vi "Send Basic Command Packet.vi"(9 "Solenoid States":bool[](array[boolean]), 11 "Output Enable":bool) -> ()   [LabVIEW 2015]
uses:
  Control Packet - Basic.ctl
  Control Packet Type.ctl
  Packet Transmitter Action.ctl
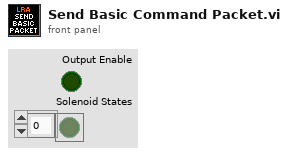
[diagram p1: front panel]
types:
  T1 = typedef "Packet Transmitter Action.ctl" = enum16{"Initialize", "Enqueue for Send", "Retrieve for Send"}
  T2 = typedef "Control Packet Type.ctl" = enum8{"Basic"}
  T3 = typedef "Control Packet - Basic.ctl" = cluster{"Solenoid Commands":bool[], "Output Enable":bool, "Timestamp":u32}
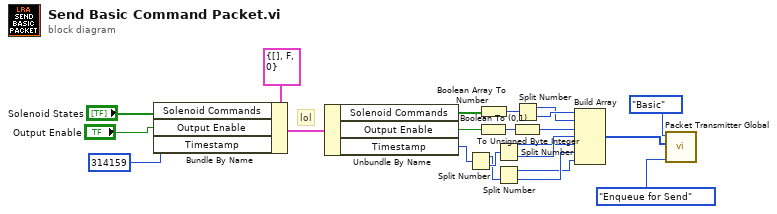
[diagram p0: block diagram]
diagram:
  # "lol"
  n1 = Bundle By Name(cluster=T3 {"Solenoid Commands"=[], "Output Enable"=FALSE, "Timestamp"=0} ("Cluster"), "Solenoid Commands"="Solenoid States", "Output Enable"="Output Enable", "Timestamp"=u32 314159) -> (w19:T3)
  n2 = Unbundle By Name(w19) -> ("Solenoid Commands"=w18:bool[], "Output Enable"=w17:bool, "Timestamp"=w11:u32)
  n3 = Split Number(x=w11) -> (hi(x)=w9:u16, lo(x)=w10:u16)
  n4 = Boolean To (0,1)(Boolean=w17) -> (0, 1=w13:i16)
  n5 = Boolean Array To Number(Boolean array=w18) -> (number=w16:u16)
  n6 = Split Number(x=w10) -> (hi(x)=w7:u8, lo(x)=w8:u8)
  n7 = Split Number(x=w9) -> (hi(x)=w5:u8, lo(x)=w6:u8)
  n8 = To Unsigned Byte Integer(number=w13) -> (unsigned 8bit integer=w12:u8)
  n9 = Split Number(x=w16) -> (hi(x)=w14:u8, lo(x)=w15:u8)
  n10 = Build Array(w15, w14, w12, w8, w7, w6, w5) -> (w4:u8[])
  n11 = call "Packet Transmitter Global.vi"("Action"=Packet_Transmitter_Action."Enqueue for Send", "Data In"=w4, "Packet Type"=Control_Packet_Type."Basic") -> ()  [unwired: 8 in, 1 out]
